vi "Tmp_M test UI.vi"() -> ()   [LabVIEW 2021, in "Magnet module.lvlib"]
uses:
  Magnet module.lvlib
  Messenger service/MessengerLib.lvlib
  submodules/Temperature monitor/Temperature monitor.lvlib
  ctl/Cryostat temperature sensors.ctl
  submodules/Temperature monitor/Typedefs/TM Revision.ctl
  Messenger service/Data types/MSG to TOP.ctl
  Messenger service/Data types/Module name.ctl
panel:
  out "data 2":T1
  in  "timeout ms":i32=2000
  out "data":T2 {"Time stamp" format="%<%H:%M:%S%2u\n%Y/%m/%d>T"}
  in  "Set timeout":bool
  in  "Force Update":bool
  in  "stop":bool
  out "MSG packet":T3
  out "Initialized":bool=TRUE
  out "Ended":bool=TRUE
  out "Temperatures":T2[](array[typedef]) {"Time stamp" format="%<%H:%M:%S%2u\n%Y/%m/%d>T"}
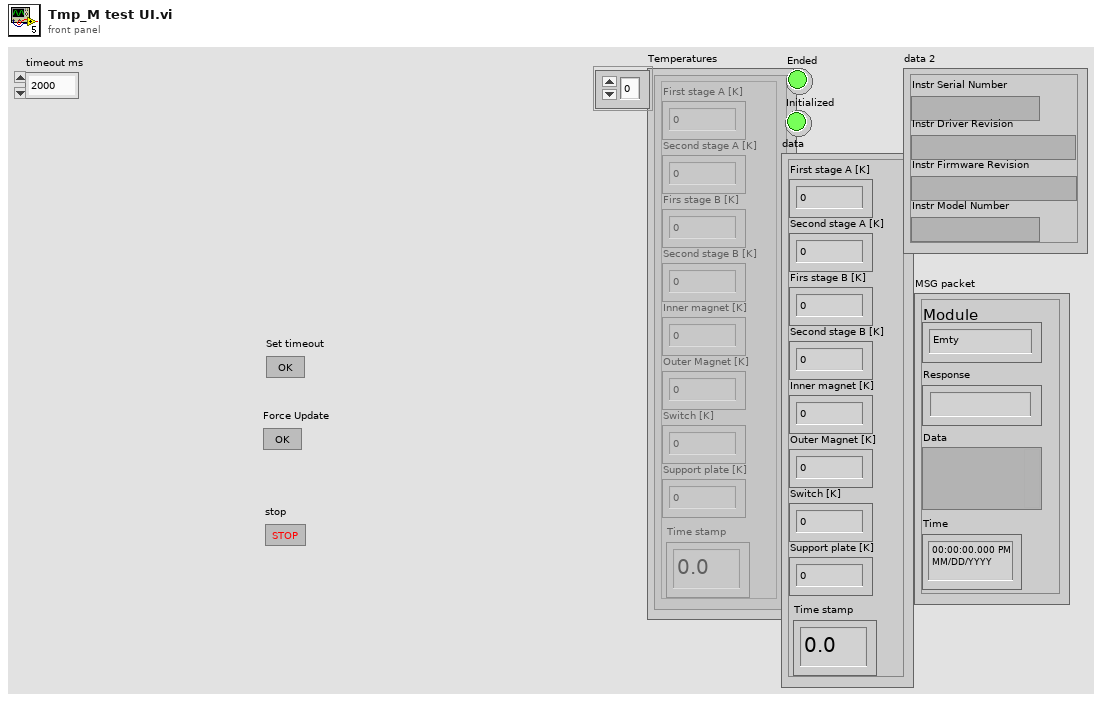
[diagram p1: front panel]
types:
  T1 = typedef "Temperature monitor.lvlib/TM Revision.ctl" = cluster{"Instr Serial Number":string, "Instr Driver Revision":string, "Instr Firmware Revision":string, "Instr Model Number":string}
  T2 = typedef "Cryostat temperature sensors.ctl" = cluster{"First stage A [K]":dbl, "Second stage A [K]":dbl, "Firs stage B [K]":dbl, "Second stage B [K]":dbl, "Inner magnet [K]":dbl, "Outer Magnet [K]":dbl, "Switch [K]":dbl, "Support plate [K]":dbl, "Time stamp":dbl}
  T3 = typedef "MessengerLib.lvlib/MSG to TOP.ctl" = cluster{"Module":T4, "Response":string, "Data":variant, "Time":timestamp}
  T4 = typedef "MessengerLib.lvlib/Module name.ctl" = enum16{"Emty", "Magnet", "VTI", "Excitation", "Servo", "Acquisition", "Rotator", "Digitizer", "SMU2450", "Carousel", "Multimeter", "Tmp monitor", "Power monitor"}
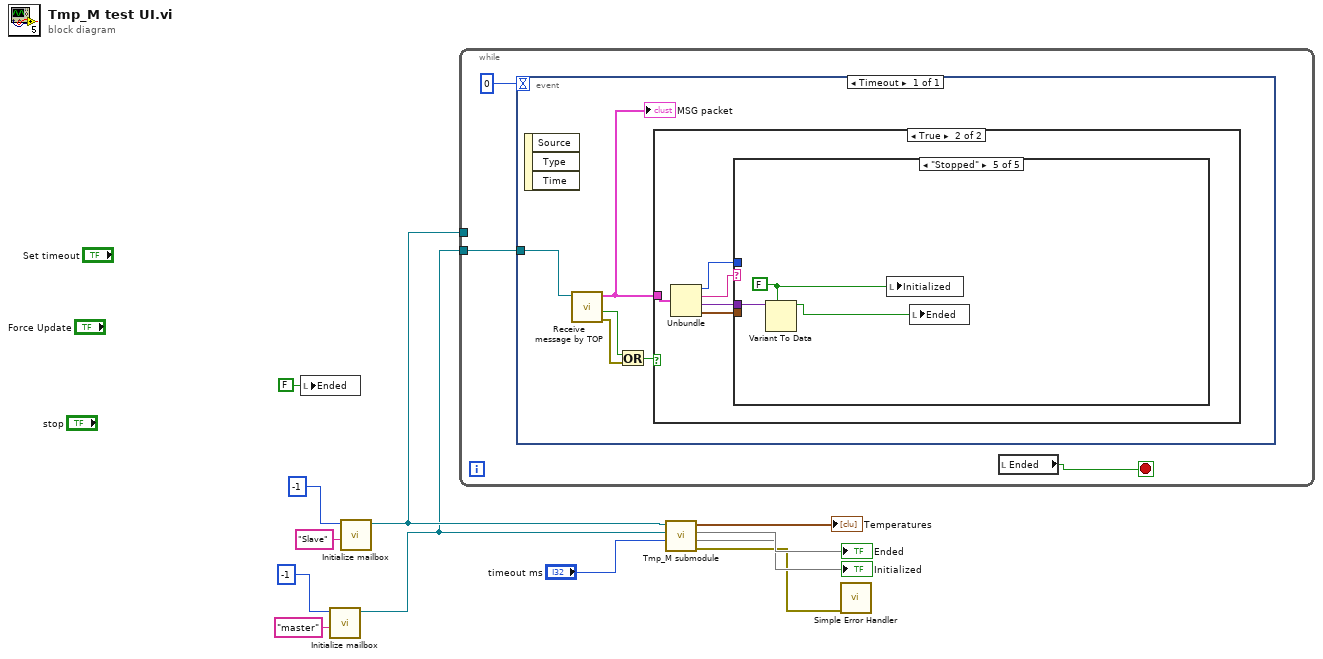
[diagram p0: block diagram]
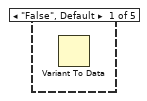
[diagram p3: hidden frame]
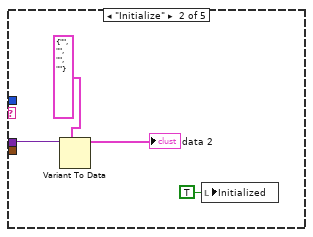
[diagram p4: hidden frame]
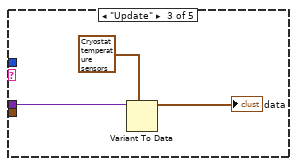
[diagram p5: hidden frame]
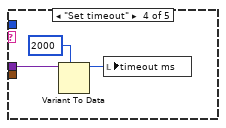
[diagram p6: hidden frame]
diagram:
  n1 = local write "Ended"(FALSE ("Ended")) -> ()
  n2 = call "Initialize mailbox.vi"("name (unnamed)"="master", "MailboxSize(-1)"=-1) -> ("Queue out"=w2:refnum<queue>)  [unwired: 8 in, 1 out]
  n3 = call "Initialize mailbox.vi"("name (unnamed)"="Slave", "MailboxSize(-1)"=-1) -> ("Queue out"=w3:refnum<queue>)  [unwired: 8 in, 1 out]
  n4 = while {
    tunnel: w3 -> [_]
    tunnel: w2 -> [w14]
    stop <- w13 stop-if-true
    n5 = event shown="[0] Timeout" {
      selector: _ -> [_]
      dyn-events: _ -> [_]
      timeout: 0 -> [_]
      tunnel: w14 -> [w20]
      event Timeout {
        n6 = event-data() -> ()  [unwired: 1 in, 3 out]
        n7 = call "Receive message by TOP.vi"("Mailbox in"=w20) -> ("error out"=w16:errorcluster, "timed out?"=w17:bool, "MSG packet"=w19:T3)  [unwired: 7 in, 1 out]
        "MSG packet" <- w19
        n8 = Or(x=w17, y=w16) -> (x .or. y?=w18:bool)
        n9 = case shown="True" w18 {
          tunnel: w19 -> [_ w25]
          frame False {
          }
          frame True {
            n10 = Unbundle(w25) -> ("Module"=w21:T4, "Response"=w24:string, "Data"=w22:variant, "Time"=w23:timestamp)
            n11 = case shown="\"Stopped\"" w24 {
              tunnel: w23 -> [_ _ _ _ _]
              tunnel: w22 -> [_ w29 w32 w35 w38]
              tunnel: w21 -> [_ _ _ _ _]
              frame "False", Default {
                n12 = Variant To Data() -> ()  [unwired: 3 in, 2 out]
              }
              frame "Initialize" {
                n13 = Variant To Data(type=T1 {"Instr Serial Number"="", "Instr Driver Revision"="", "Instr Firmware Revision"="", "Instr Model Number"=""} ("TM Revision"), Variant=w29) -> (data=→"data 2":T1)  [unwired: 1 in, 1 out]
                n14 = local write "Initialized"(TRUE ("Initialized")) -> ()
              }
              frame "Update" {
                n15 = Variant To Data(type=T2 {"First stage A [K]"=0.0, "Second stage A [K]"=0.0, "Firs stage B [K]"=0.0, "Second stage B [K]"=0.0, "Inner magnet [K]"=0.0, "Outer Magnet [K]"=0.0, "Switch [K]"=0.0, "Support plate [K]"=0.0, "Time stamp"=0.0} ("LSC218 sensors"), Variant=w32) -> (data=→"data":T2)  [unwired: 1 in, 1 out]
              }
              frame "Set timeout" {
                n16 = Variant To Data(type=2000 ("timeout ms"), Variant=w35) -> (data=w33:i32)  [unwired: 1 in, 1 out]
                n17 = local write "timeout ms"(w33) -> ()
              }
              frame "Stopped" {
                w36 = FALSE ("Initialized 2")
                n18 = Variant To Data(type=w36, Variant=w38) -> (data=w37:bool)  [unwired: 1 in, 1 out]
                n19 = local write "Initialized"(w36) -> ()
                n20 = local write "Ended"(w37) -> ()
              }
            }
          }
        }
      }
    }
    n21 = local read "Ended"() -> (w13:bool)
  }
  n22 = call "Tmp_M submodule.vi"(9:"timeout ms", 10:w2, 11:w3) -> ("Error Out"=w5:errorcluster, 1:→"Initialized", 2:→"Ended", "Temperatures"=→"Temperatures":T2[])  [unwired: 5 in]
  n23 = call <vilib>:"Simple Error Handler.vi"("error in (no error)"=w5) -> ()  [unwired: 4 in, 5 out]
